vi "LoggingProcess.vi"(0 "FPGA Interface":refnum<k20>, 5 "Buffers":T2={"Channels"=[], "PosttriggerBuffer"=refnum, "PretriggerBuffer"=refnum, "BlockSizePerChannel"=0, " logging semaphore"=refnum, "Log refnum"=refnum, "snapshotBuffer"=refnum, "logDirectory"=path "", "logPrefix"="", "decimation factor"=1, "max files"=0, "SampleRate"=0.0}, 7 "WaveformConfiguration":T1, 11 "error in (no error)":errorcluster) -> ()   [LabVIEW 2017]
uses:
  <vilib>/NI/PowerElectronicsControl/BufferLogging/Buffers.ctl
  <vilib>/NI/DCAF/Modules/FPGAWaveform/execution/Export.ctl
  FPGA/FPGAtypedef.ctl
  globals.vi
  <vilib>/Utility/error.llb/Error Cluster From Error Code.vi
  <vilib>/RVI Host/nirviSupport.llb/nirviErrorClusterFromErrorCode.vi
  <vilib>/rvi/errors/niLvFpgaAdjustHostInterfaceError.vi
  <vilib>/rvi/interface/nirviMethod/nirviMethod.xnode
  <vilib>/rvi/interface/nirviReadWriteControl/nirviReadWriteControl.xnode
  <vilib>/NI/PowerElectronicsControl/BufferLogging/BufferLogging.lvlib
  <vilib>/rvi/interface/nirviMethod/StockFPGA_InlinedMethodWaitForSingleIRQ.vi
  <vilib>/FPGAPlugInAG/Dynamic/niLvFpga_WaitOnIrq_Dynamic.vi
  <vilib>/FPGAPlugInAG/Dynamic/niLvFpga_AcknowledgeIrq_Dynamic.vi
  NiFpgaLv.dll
  <vilib>/rvi/interface/Simulation/niFpgaSimulationCallBeginRW.vi
  <vilib>/NI/DCAF/Modules/FPGAWaveform/execution/WaveformAcq runtime.lvclass
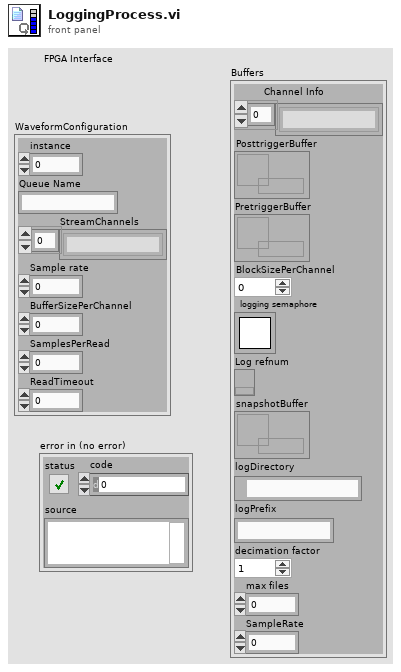
[diagram p1: front panel]
types:
  T1 = typedef "WaveformAcq runtime.lvclass/Export.ctl" = cluster{"instance":i32, "Queue Name":string, "StreamChannels":string[], "Sample rate":i32, "BufferSizePerChannel":i32, "SamplesPerRead":i32, "ReadTimeout":dbl}
  T2 = typedef "BufferLogging.lvlib/Buffers.ctl" = cluster{"Channels":string[], "PosttriggerBuffer":refnum<queue>, "PretriggerBuffer":refnum<queue>, "BlockSizePerChannel":i32, " logging semaphore":T3, "Log refnum":refnum<k34>, "snapshotBuffer":refnum<data-value>, "logDirectory":path, "logPrefix":string, "decimation factor":i32, "max files":i32, "SampleRate":dbl}
  T3 = typedef "Semaphore RefNum" = refnum<k1>
  T4 = typedef "FPGAtypedef.ctl" = refnum<k20>
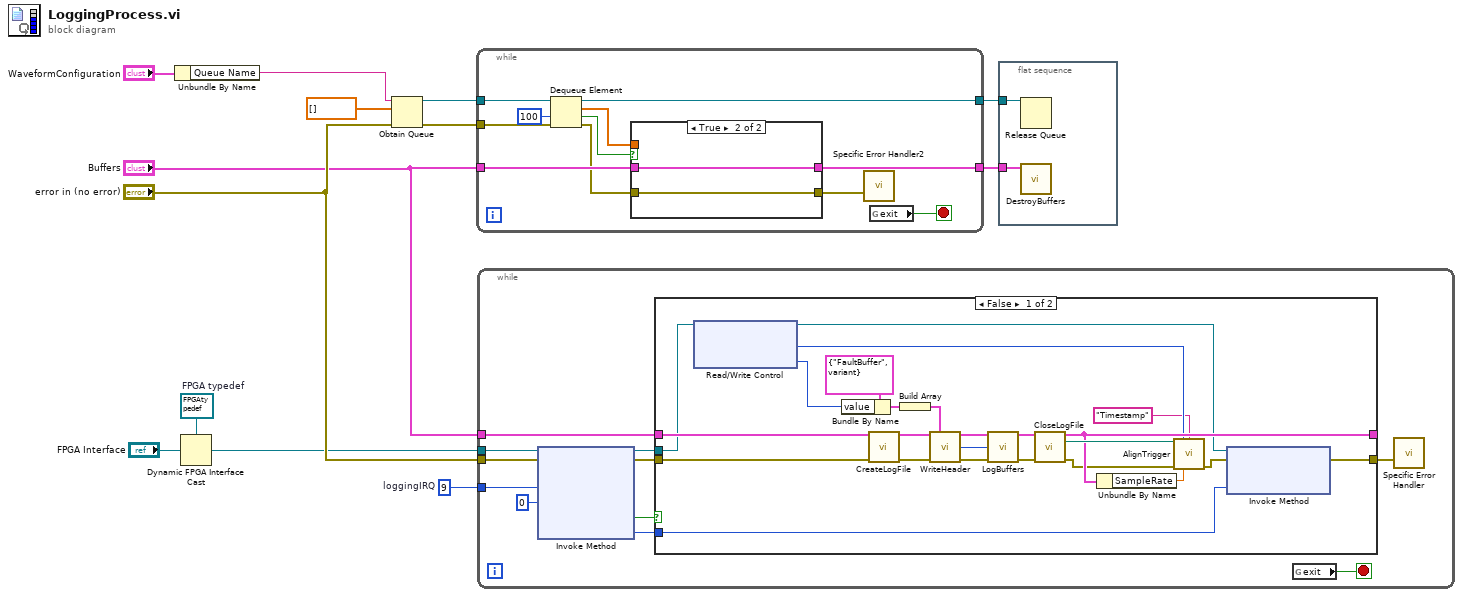
[diagram p0: block diagram]
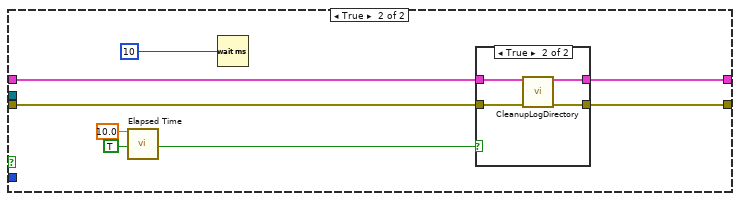
[diagram p2: hidden frame]
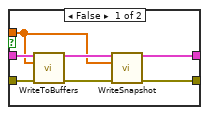
[diagram p4: hidden frame]
diagram:
  w1 = T4 refnum  # FPGA typedef
  w8 = 9  # loggingIRQ
  n1 = Unbundle By Name("WaveformConfiguration") -> ("Queue Name"=w4:string)
  n2 = Dynamic FPGA Interface Cast(Session In=w1, Type="FPGA Interface") -> (Session Out=w2:T4)
  n3 = Obtain Queue(name (unnamed)=w4, element data type=sgl[] [], error in (no error)="error in (no error)") -> (queue out=w11:refnum<queue>, error out=w12:errorcluster)  [unwired: 2 in, 1 out]
  n4 = while {
    tunnel: w11 -> [w24]
    tunnel: w12 -> [w23]
    tunnel: [w21] -> w13
    tunnel: "Buffers" -> [w19]
    tunnel: [w15] -> w9
    stop <- w20 stop-if-true
    n5 = Dequeue Element(queue=w24, timeout in ms (-1)=100, error in (no error)=w23) -> (queue out=w21:refnum<queue>, element=w16:sgl[], timed out?=w17:bool, error out=w18:errorcluster)
    n6 = case shown="True" w17 {
      tunnel: w19 -> [w30 w32]
      tunnel: w18 -> [w29 w33]
      tunnel: [w27 w33] -> w14
      tunnel: w16 -> [w26 _]
      tunnel: [w25 w32] -> w15
      frame False {
        n7 = call <vilib>:"WriteToBuffers.vi"("Buffers in"=w30, "Data"=w26, "error in (no error)"=w29) -> ("Buffers out"=w31:T2, "error out"=w28:errorcluster)  [unwired: 11 in]
        n8 = call <vilib>:"WriteSnapshot.vi"("Buffers in"=w31, "Snapshot"=w26, "error in (no error)"=w28) -> ("Buffers out"=w25:T2, "error out"=w27:errorcluster)  [unwired: 11 in]
      }
      frame True {
      }
    }
    n9 = call "Specific Error Handler2"("Error to Check"=w14) -> ()  [unwired: 11 in, 4 out]
    n10 = global read "globals.vi" "exit"() -> (w20:bool)
  }
  n11 = while {
    tunnel: "error in (no error)" -> [w40]
    tunnel: "Buffers" -> [w42]
    tunnel: w2 -> [w43]
    tunnel: w8 -> [w41]
    stop <- w44 stop-if-true
    n12 = xnode "Invoke Method"("FPGA VI Reference In"=w43, "error in"=w40, "IRQ Number(s)"=w41, "Timeout (ms)"=0) -> ("FPGA VI Reference Out"=w36:T4, "error out"=w39:errorcluster, "Timed Out"=w37:bool, "IRQ(s) Asserted"=w35:i32)
    n13 = case shown="False" w37 {
      tunnel: w39 -> [w59 w72]
      tunnel: w42 -> [w68 w70]
      tunnel: [w54 w69] -> _
      tunnel: [w60 w71] -> w34
      tunnel: w36 -> [w55 _]
      tunnel: w35 -> [w58 _]
      frame False {
        n14 = xnode "Read/Write Control"("FPGA VI Reference In"=w55) -> ("FPGA VI Reference Out"=w52:T4, "TriggerTimestamp"=w51:i32, "FaultBuffer"=w48:u64)  [unwired: 1 in, 1 out]
        n15 = Bundle By Name(cluster=cluster{"Property":string, "value":variant} {"Property"="FaultBuffer", "value"=variant}, "value"=w48) -> (w47:cluster{"Property":string, "value":variant})
        n16 = call <vilib>:"CreateLogFile.vi"("Buffers in"=w68, "error in (no error)"=w59) -> ("Buffers out"=w67:T2, "error out"=w66:errorcluster)  [unwired: 12 in]
        n17 = Build Array(w47) -> (w46:cluster{"Property":string, "value":variant}[])
        n18 = call <vilib>:"WriteHeader.vi"("Buffers in"=w67, "LogMetaData"=w46, "error in (no error)"=w66) -> ("Buffers out"=w65:T2, "numOfChannels"=w63:i32, "error out"=w64:errorcluster)  [unwired: 10 in]
        n19 = call <vilib>:"LogBuffers.vi"("Buffers in"=w65, "numOfChannels"=w63, "error in (no error)"=w64) -> ("Buffers out"=w62:T2, "error out"=w61:errorcluster)  [unwired: 11 in]
        n20 = call <vilib>:"CloseLogFile.vi"("Buffers in"=w62, "error in (no error)"=w61) -> ("Buffers out"=w54:T2, "log path out"=w57:path, "error out"=w50:errorcluster)  [unwired: 11 in]
        n21 = Unbundle By Name(w54) -> ("SampleRate"=w53:dbl)
        n22 = call <vilib>:"AlignTrigger.vi"("log path in"=w57, "triggerTimestamp"=w51, "alignmentChannel"="Timestamp", "error in (no error)"=w50, "AcqRate"=w53) -> ("error out"=w56:errorcluster)  [unwired: 9 in, 1 out]
        n23 = xnode "Invoke Method"("FPGA VI Reference In"=w52, "error in"=w56, "IRQ Number(s)"=w58) -> ("error out"=w60:errorcluster)  [unwired: 1 out]
      }
      frame True {
        n24 = call "Elapsed Time"("Time Target (s)"=10.0, "Auto Reset"=TRUE) -> ("Time has Elapsed"=w73:bool)  [unwired: 10 in, 7 out]
        n25 = Wait (ms)(milliseconds to wait=u32 10) -> ()  [unwired: 1 out]
        n26 = case shown="True" w73 {
          tunnel: w72 -> [w78 w82]
          tunnel: [w78 w81] -> w71
          tunnel: w70 -> [w77 w80]
          tunnel: [w77 w79] -> w69
          frame False {
          }
          frame True {
            n27 = call <vilib>:"CleanupLogDirectory.vi"("BuffersIn"=w80, "error in"=w82) -> ("BuffersOut"=w79:T2, "error out"=w81:errorcluster)  [unwired: 12 in]
          }
        }
      }
    }
    n28 = global read "globals.vi" "exit"() -> (w44:bool)
    n29 = call "Specific Error Handler"("Error to Check"=w34) -> ()  [unwired: 11 in, 4 out]
  }
  n30 = flat-sequence {
    tunnel: w13 -> [w84]
    tunnel: w9 -> [w83]
    frame #0 {
      n31 = Release Queue(queue=w84) -> ()  [unwired: 2 in, 3 out]
      n32 = call <vilib>:"DestroyBuffers.vi"("Buffers"=w83) -> ()  [unwired: 14 in, 1 out]
    }
  }
